vi "Shutdown.vi"(8 "error in (no error)":errorcluster, 11 "Modbus slave in":refnum<class "Modbus Slave.lvclass">) -> (0 "error out":errorcluster)   [LabVIEW 2021, in "Modbus Slave.lvclass"]
doc: "Closes and destroys a Modbus slave instance."
uses:
  Modbus Slave.lvclass
  Modbus Slave.lvclass/Modbus Slave.ctl
  Network Protocol/Network Slave/Network Slave.lvclass
  Data Model/Device Data Model.lvclass
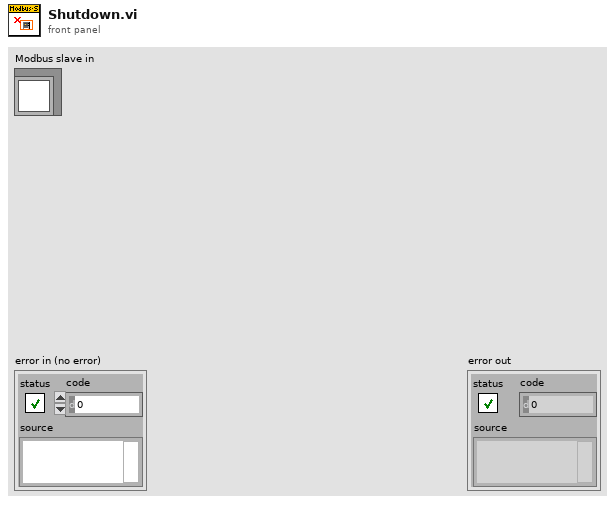
[diagram p1: front panel]
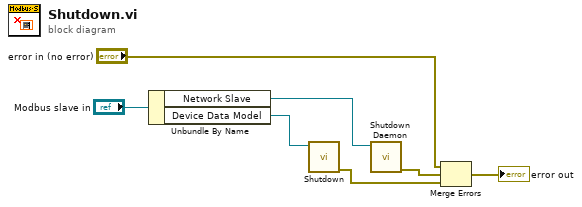
[diagram p0: block diagram]
diagram:
  n1 = Unbundle By Name("Modbus slave in") -> ("Network Slave"=w1:refnum<class "Network Slave.lvclass">, "Device Data Model"=w7:refnum<class "Device Data Model.lvclass">)
  n2 = call-dynamic "Shutdown.vi"("device data model in"=w7) -> ("error out"=w2:errorcluster)  [unwired: 10 in]
  n3 = call-dynamic "Shutdown Daemon.vi"("network slave in"=w1) -> ("error out"=w3:errorcluster)  [unwired: 10 in]
  n4 = Merge Errors("error in (no error)", w3, w2) -> (→"error out":errorcluster)
